vi "Spectral Leakage & window effect.vi"() -> ()   [LabVIEW 2009]
uses:
  <vilib>/Analysis/2dsp.llb/Power Spectrum (DBL).vi
  <vilib>/Analysis/4window.llb/Hanning Window (DBL).vi
  <vilib>/Analysis/4window.llb/Hamming Window (DBL).vi
  <vilib>/Analysis/4window.llb/Triangle Window (DBL).vi
  <vilib>/Analysis/4window.llb/Exponential Window (DBL).vi
  <vilib>/Analysis/4window.llb/Kaiser-Bessel Window (DBL).vi
  <vilib>/Analysis/NI_AALBase.lvlib
  <vilib>/Analysis/NI_AALPro.lvlib
panel:
  out "?":bool
  out "Time domain waveform with periodic repetition":dbl[](graph)=[0.0, 0.06279051952931337, 0.12533323356430423, 0.18738131458572463, 0.24868988716485477, 0.3090169943749474, 0.3681245526846779, 0.42577929156507266, 0.48175367410171527, 0.5358267949789965, 0.5877852522924731, 0.6374239897486896, 0.6845471059286886, 0.7289686274214116, 0.7705132427757893, 0.8090169943749475, 0.8443279255020151, 0.8763066800438636, 0.9048270524660195, 0.9297764858882513, 0.9510565162951535, 0.9685831611286311, 0.9822872507286887, 0.9921147013144779, 0.9980267284282716, 1.0, 0.9980267284282716, 0.9921147013144779, 0.9822872507286887, 0.9685831611286312, 0.9510565162951536, 0.9297764858882515, 0.9048270524660196, 0.8763066800438636, 0.8443279255020151, 0.8090169943749475, 0.7705132427757893, 0.7289686274214116, 0.6845471059286887, 0.6374239897486897, 0.5877852522924732, 0.5358267949789967, 0.4817536741017154, 0.42577929156507277, 0.3681245526846781, 0.3090169943749475, 0.2486898871648549, 0.18738131458572474, 0.12533323356430437, 0.0627905195293135, 1.2354483755472323e-16, -0.06279051952931325, -0.12533323356430412, -0.1873813145857245, -0.24868988716485466, -0.3090169943749473, -0.3681245526846778, -0.42577929156507255, -0.48175367410171516, -0.5358267949789965, -0.587785252292473, -0.6374239897486896, -0.6845471059286886, -0.7289686274214114, -0.7705132427757891, -0.8090169943749473, -0.844327925502015, -0.8763066800438635, -0.9048270524660195, -0.9297764858882513, -0.9510565162951535, -0.9685831611286311, -0.9822872507286886, -0.9921147013144778, -0.9980267284282716, -1.0, -0.9980267284282716, -0.9921147013144779, -0.9822872507286887, -0.9685831611286312, -0.9510565162951536, -0.9297764858882515, -0.9048270524660196, -0.8763066800438637, -0.8443279255020152, -0.8090169943749476, -0.7705132427757894, -0.7289686274214117, -0.6845471059286888, -0.6374239897486899, -0.5877852522924734, -0.5358267949789968, -0.4817536741017155, -0.4257792915650729, -0.3681245526846782, -0.3090169943749477, -0.24868988716485502, -0.18738131458572488, -0.12533323356430448, -0.06279051952931362, 0.0, 0.06279051952931337, 0.12533323356430423, 0.18738131458572463, 0.24868988716485477, 0.3090169943749474, 0.3681245526846779, 0.42577929156507266, 0.48175367410171527, 0.5358267949789965, 0.5877852522924731, 0.6374239897486896, 0.6845471059286886, 0.7289686274214116, 0.7705132427757893, 0.8090169943749475, 0.8443279255020151, 0.8763066800438636, 0.9048270524660195, 0.9297764858882513, 0.9510565162951535, 0.9685831611286311, 0.9822872507286887, 0.9921147013144779, 0.9980267284282716, 1.0, 0.9980267284282716, 0.9921147013144779, 0.9822872507286887, 0.9685831611286312, 0.9510565162951536, 0.9297764858882515, 0.9048270524660196, 0.8763066800438636, 0.8443279255020151, 0.8090169943749475, 0.7705132427757893, 0.7289686274214116, 0.6845471059286887, 0.6374239897486897, 0.5877852522924732, 0.5358267949789967, 0.4817536741017154, 0.42577929156507277, 0.3681245526846781, 0.3090169943749475, 0.2486898871648549, 0.18738131458572474, 0.12533323356430437, 0.0627905195293135, 1.2354483755472323e-16, -0.06279051952931325, -0.12533323356430412, -0.1873813145857245, -0.24868988716485466, -0.3090169943749473, -0.3681245526846778, -0.42577929156507255, -0.48175367410171516, -0.5358267949789965, -0.587785252292473, -0.6374239897486896, -0.6845471059286886, -0.7289686274214114, -0.7705132427757891, -0.8090169943749473, -0.844327925502015, -0.8763066800438635, -0.9048270524660195, -0.9297764858882513, -0.9510565162951535, -0.9685831611286311, -0.9822872507286886, -0.9921147013144778, -0.9980267284282716, -1.0, -0.9980267284282716, -0.9921147013144779, -0.9822872507286887, -0.9685831611286312, -0.9510565162951536, -0.9297764858882515, -0.9048270524660196, -0.8763066800438637, -0.8443279255020152, -0.8090169943749476, -0.7705132427757894, -0.7289686274214117, -0.6845471059286888, -0.6374239897486899, -0.5877852522924734, -0.5358267949789968, -0.4817536741017155, -0.4257792915650729, -0.3681245526846782, -0.3090169943749477, -0.24868988716485502, -0.18738131458572488, -0.12533323356430448, -0.06279051952931362, 0.0, 0.06279051952931337, 0.12533323356430423, 0.18738131458572463, 0.24868988716485477, 0.3090169943749474, 0.3681245526846779, 0.42577929156507266, 0.48175367410171527, 0.5358267949789965, 0.5877852522924731, 0.6374239897486896, 0.6845471059286886, 0.7289686274214116, 0.7705132427757893, 0.8090169943749475, 0.8443279255020151, 0.8763066800438636, 0.9048270524660195, 0.9297764858882513, 0.9510565162951535, 0.9685831611286311, 0.9822872507286887, 0.9921147013144779, 0.9980267284282716, 1.0, 0.9980267284282716, 0.9921147013144779, 0.9822872507286887, 0.9685831611286312, 0.9510565162951536, 0.9297764858882515, 0.9048270524660196, 0.8763066800438636, 0.8443279255020151, 0.8090169943749475, 0.7705132427757893, 0.7289686274214116, 0.6845471059286887, 0.6374239897486897, 0.5877852522924732, 0.5358267949789967, 0.4817536741017154, 0.42577929156507277, 0.3681245526846781, 0.3090169943749475, 0.2486898871648549, 0.18738131458572474, 0.12533323356430437, 0.0627905195293135, 1.2354483755472323e-16, -0.06279051952931325, -0.12533323356430412, -0.1873813145857245, -0.24868988716485466, -0.3090169943749473, -0.3681245526846778, -0.42577929156507255, -0.48175367410171516, -0.5358267949789965, -0.587785252292473, -0.6374239897486896, -0.6845471059286886, -0.7289686274214114, -0.7705132427757891, -0.8090169943749473, -0.844327925502015, -0.8763066800438635, -0.9048270524660195, -0.9297764858882513, -0.9510565162951535, -0.9685831611286311, -0.9822872507286886, -0.9921147013144778, -0.9980267284282716, -1.0, -0.9980267284282716, -0.9921147013144779, -0.9822872507286887, -0.9685831611286312, -0.9510565162951536, -0.9297764858882515, -0.9048270524660196, -0.8763066800438637, -0.8443279255020152, -0.8090169943749476, -0.7705132427757894, -0.7289686274214117, -0.6845471059286888, -0.6374239897486899, -0.5877852522924734, -0.5358267949789968, -0.4817536741017155, -0.4257792915650729, -0.3681245526846782, -0.3090169943749477, -0.24868988716485502, -0.18738131458572488, -0.12533323356430448, -0.06279051952931362]
  in  "Beta":dbl
  in  "Final value":dbl min=0.0 max=1.0
  in  "WINDOW SELECTION":T1(ring)
  out "Frequency\n Domain (without Nyquist shift)":cluster{dbl[]}[](graph)=[{[-717.9728168160375, -12.041199826559248, -665.4873643647093, -666.5995099029594, -669.1691632658144, -677.6948998948894, -681.0329352713741, -671.6665379094907, -689.1835321816163, -671.0719482760868, -689.2418614836788, -672.621826473416, -701.957270271522, -696.8532852986106, -699.451463656731, -692.8383353860734, -682.2898330103367, -698.4054730062687, -707.0532336610472, -669.1255959463351, -707.2021141139068, -686.286325714701, -709.9481162420018, -722.3894498312288, -680.343553829749, -707.4833793420511, -683.1290877804176, -715.3954757206127, -701.1845387253027, -662.9236503342374, -702.6771685318919, -678.1983559742026, -688.0233871040186, -694.8478727739428, -682.6498613386614, -710.6827112012634, -685.7413183239719, -695.7380708290177, -702.9080625621561, -687.1093940743207, -701.1813999614833, -687.5117716388966, -683.6478766075195, -693.9397092458923, -696.0469234579446, -697.7718028900654, -700.095895469833, -691.0074396642474, -694.6133804341445, -703.2922193198955, -697.7736277833116, -703.2922193198955, -694.6133804341445, -691.0074396642474, -700.095895469833, -697.7718028900654, -696.0469234579446, -693.9397092458923, -683.6478766075195, -687.5117716388966, -701.1813999614833, -687.1093940743207, -702.9080625621561, -695.7380708290177, -685.7413183239719, -710.6827112012634, -682.6498613386614, -694.8478727739428, -688.0233871040186, -678.1983559742026, -702.6771685318919, -662.9236503342374, -701.1845387253027, -715.3954757206127, -683.1290877804176, -707.4833793420511, -680.343553829749, -722.3894498312288, -709.9481162420018, -686.286325714701, -707.2021141139068, -669.1255959463351, -707.0532336610472, -698.4054730062687, -682.2898330103367, -692.8383353860734, -699.451463656731, -696.8532852986106, -701.957270271522, -672.621826473416, -689.2418614836788, -671.0719482760868, -689.1835321816163, -671.6665379094907, -681.0329352713741, -677.6948998948894, -669.1691632658144, -666.5995099029594, -665.4873643647093, -12.041199826559248]}, {[-662.5234612067311, -24.082399653118497, -36.12359947967774, -686.0391501168739, -674.2650878771286, -705.9966216646466, -682.162384061586, -693.5568602960511, -708.2455189374288, -676.9926374665027, -713.7575746206643, -678.0624747732352, -692.8167424503345, -688.5243172746942, -693.2645231323679, -701.7444563843032, -695.9087779401403, -690.0885198379467, -690.4467642576584, -682.1856808023391, -728.2256383540973, -683.3629541008854, -687.4572822103436, -724.8745272591966, -713.4517040919175, -703.5234323149774, -698.75063890254, -693.7459180991335, -696.0122919812911, -673.7183454293233, -693.9731458975725, -677.0281334674862, -712.0669993234728, -722.7708351339987, -688.1087311691958, -699.2377312537521, -705.1978959578129, -697.4552667133765, -715.643610874567, -694.98626076297, -731.5654873669778, -685.4026578115215, -694.3961609277321, -718.8382831595254, -691.9463362592454, -697.3136367707239, -761.427863621243, -702.8552652123016, -688.0472344934774, -705.6030194961304, -708.6337726784353, -705.6030194961304, -688.0472344934774, -702.8552652123016, -761.427863621243, -697.3136367707239, -691.9463362592454, -718.8382831595254, -694.3961609277321, -685.4026578115215, -731.5654873669778, -694.98626076297, -715.643610874567, -697.4552667133765, -705.1978959578129, -699.2377312537521, -688.1087311691958, -722.7708351339987, -712.0669993234728, -677.0281334674862, -693.9731458975725, -673.7183454293233, -696.0122919812911, -693.7459180991335, -698.75063890254, -703.5234323149774, -713.4517040919175, -724.8745272591966, -687.4572822103436, -683.3629541008854, -728.2256383540973, -682.1856808023391, -690.4467642576584, -690.0885198379467, -695.9087779401403, -701.7444563843032, -693.2645231323679, -688.5243172746942, -692.8167424503345, -678.0624747732352, -713.7575746206643, -676.9926374665027, -708.2455189374288, -693.5568602960511, -682.162384061586, -705.9966216646466, -674.2650878771286, -686.0391501168739, -36.12359947967774, -24.082399653118497]}]
  out "Time domain waveform":dbl[](graph)=[0.0, 0.06279051952931337, 0.12533323356430423, 0.18738131458572463, 0.24868988716485477, 0.3090169943749474, 0.3681245526846779, 0.42577929156507266, 0.48175367410171527, 0.5358267949789965, 0.5877852522924731, 0.6374239897486896, 0.6845471059286886, 0.7289686274214116, 0.7705132427757893, 0.8090169943749475, 0.8443279255020151, 0.8763066800438636, 0.9048270524660195, 0.9297764858882513, 0.9510565162951535, 0.9685831611286311, 0.9822872507286887, 0.9921147013144779, 0.9980267284282716, 1.0, 0.9980267284282716, 0.9921147013144779, 0.9822872507286887, 0.9685831611286312, 0.9510565162951536, 0.9297764858882515, 0.9048270524660196, 0.8763066800438636, 0.8443279255020151, 0.8090169943749475, 0.7705132427757893, 0.7289686274214116, 0.6845471059286887, 0.6374239897486897, 0.5877852522924732, 0.5358267949789967, 0.4817536741017154, 0.42577929156507277, 0.3681245526846781, 0.3090169943749475, 0.2486898871648549, 0.18738131458572474, 0.12533323356430437, 0.0627905195293135, 1.2354483755472323e-16, -0.06279051952931325, -0.12533323356430412, -0.1873813145857245, -0.24868988716485466, -0.3090169943749473, -0.3681245526846778, -0.42577929156507255, -0.48175367410171516, -0.5358267949789965, -0.587785252292473, -0.6374239897486896, -0.6845471059286886, -0.7289686274214114, -0.7705132427757891, -0.8090169943749473, -0.844327925502015, -0.8763066800438635, -0.9048270524660195, -0.9297764858882513, -0.9510565162951535, -0.9685831611286311, -0.9822872507286886, -0.9921147013144778, -0.9980267284282716, -1.0, -0.9980267284282716, -0.9921147013144779, -0.9822872507286887, -0.9685831611286312, -0.9510565162951536, -0.9297764858882515, -0.9048270524660196, -0.8763066800438637, -0.8443279255020152, -0.8090169943749476, -0.7705132427757894, -0.7289686274214117, -0.6845471059286888, -0.6374239897486899, -0.5877852522924734, -0.5358267949789968, -0.4817536741017155, -0.4257792915650729, -0.3681245526846782, -0.3090169943749477, -0.24868988716485502, -0.18738131458572488, -0.12533323356430448, -0.06279051952931362]
  in  "Cycles":dbl(knob)=1.0 scale=0.0..10.0 scale format="%#.2p"
  in  "stop":bool
  out "Frequency\n Domain (with Nyquist shift)":cluster{dbl[]}[](graph)=[{[-697.7736277833116, -703.2922193198955, -694.6133804341445, -691.0074396642474, -700.095895469833, -697.7718028900654, -696.0469234579446, -693.9397092458923, -683.6478766075195, -687.5117716388966, -701.1813999614833, -687.1093940743207, -702.9080625621561, -695.7380708290177, -685.7413183239719, -710.6827112012634, -682.6498613386614, -694.8478727739428, -688.0233871040186, -678.1983559742026, -702.6771685318919, -662.9236503342374, -701.1845387253027, -715.3954757206127, -683.1290877804176, -707.4833793420511, -680.343553829749, -722.3894498312288, -709.9481162420018, -686.286325714701, -707.2021141139068, -669.1255959463351, -707.0532336610472, -698.4054730062687, -682.2898330103367, -692.8383353860734, -699.451463656731, -696.8532852986106, -701.957270271522, -672.621826473416, -689.2418614836788, -671.0719482760868, -689.1835321816163, -671.6665379094907, -681.0329352713741, -677.6948998948894, -669.1691632658144, -666.5995099029594, -665.4873643647093, -12.041199826559248, -717.9728168160375, -12.041199826559248, -665.4873643647093, -666.5995099029594, -669.1691632658144, -677.6948998948894, -681.0329352713741, -671.6665379094907, -689.1835321816163, -671.0719482760868, -689.2418614836788, -672.621826473416, -701.957270271522, -696.8532852986106, -699.451463656731, -692.8383353860734, -682.2898330103367, -698.4054730062687, -707.0532336610472, -669.1255959463351, -707.2021141139068, -686.286325714701, -709.9481162420018, -722.3894498312288, -680.343553829749, -707.4833793420511, -683.1290877804176, -715.3954757206127, -701.1845387253027, -662.9236503342374, -702.6771685318919, -678.1983559742026, -688.0233871040186, -694.8478727739428, -682.6498613386614, -710.6827112012634, -685.7413183239719, -695.7380708290177, -702.9080625621561, -687.1093940743207, -701.1813999614833, -687.5117716388966, -683.6478766075195, -693.9397092458923, -696.0469234579446, -697.7718028900654, -700.095895469833, -691.0074396642474, -694.6133804341445, -703.2922193198955]}, {[-708.6337726784353, -705.6030194961304, -687.0278840301485, -702.8552652123016, -761.427863621243, -697.3136367707239, -691.9463362592454, -718.8382831595254, -694.3961609277321, -685.4026578115215, -731.5654873669778, -694.98626076297, -715.643610874567, -697.4552667133765, -705.1978959578129, -699.2377312537521, -688.1087311691958, -722.7708351339987, -712.0669993234728, -677.0281334674862, -693.9731458975725, -673.7183454293233, -696.0122919812911, -693.7459180991335, -698.75063890254, -703.5234323149774, -713.4517040919175, -724.8745272591966, -687.4572822103436, -683.3629541008854, -728.2256383540973, -682.1856808023391, -690.4467642576584, -690.0885198379467, -695.9087779401403, -701.7444563843032, -693.2645231323679, -688.5243172746942, -692.8167424503345, -678.0624747732352, -713.7575746206643, -676.9926374665027, -708.2455189374288, -693.5568602960511, -682.162384061586, -705.9966216646466, -674.2650878771286, -686.0391501168739, -36.12359947967774, -24.082399653118497, -662.5234612067311, -24.082399653118497, -36.12359947967774, -686.0391501168739, -674.2650878771286, -705.9966216646466, -682.162384061586, -693.5568602960511, -708.2455189374288, -676.9926374665027, -713.7575746206643, -678.0624747732352, -692.8167424503345, -688.5243172746942, -693.2645231323679, -701.7444563843032, -695.9087779401403, -690.0885198379467, -690.4467642576584, -682.1856808023391, -728.2256383540973, -683.3629541008854, -687.4572822103436, -724.8745272591966, -713.4517040919175, -703.5234323149774, -698.75063890254, -693.7459180991335, -696.0122919812911, -673.7183454293233, -693.9731458975725, -677.0281334674862, -712.0669993234728, -722.7708351339987, -688.1087311691958, -699.2377312537521, -705.1978959578129, -697.4552667133765, -715.643610874567, -694.98626076297, -731.5654873669778, -685.4026578115215, -694.3961609277321, -718.8382831595254, -691.9463362592454, -697.3136367707239, -761.427863621243, -702.8552652123016, -687.0278840301485, -705.6030194961304]}]
  # "The DFT/FFT assumes that the finite time waveform that you obtain is one period of a periodic signal that exist for all\ntime. This assumption of periodicity could result in discontinuities  in the periodic signal  & give rise to spectral leakage,\nwhereby the energy  at a  particular frequency leaks throughout the spectrum.  To reduce  the spectral  leakage, the \nfinite time waveform is multiplied by a \"window\" function."
  # "SPECTRAL LEAKAGE"
  # "WINDOW CHARACTERISTICS"
  # "EXPONENTIAL"
  # "db"
  # "db"
  # "KAISER-BESSEL"
  # "POWER SPECTRUM"
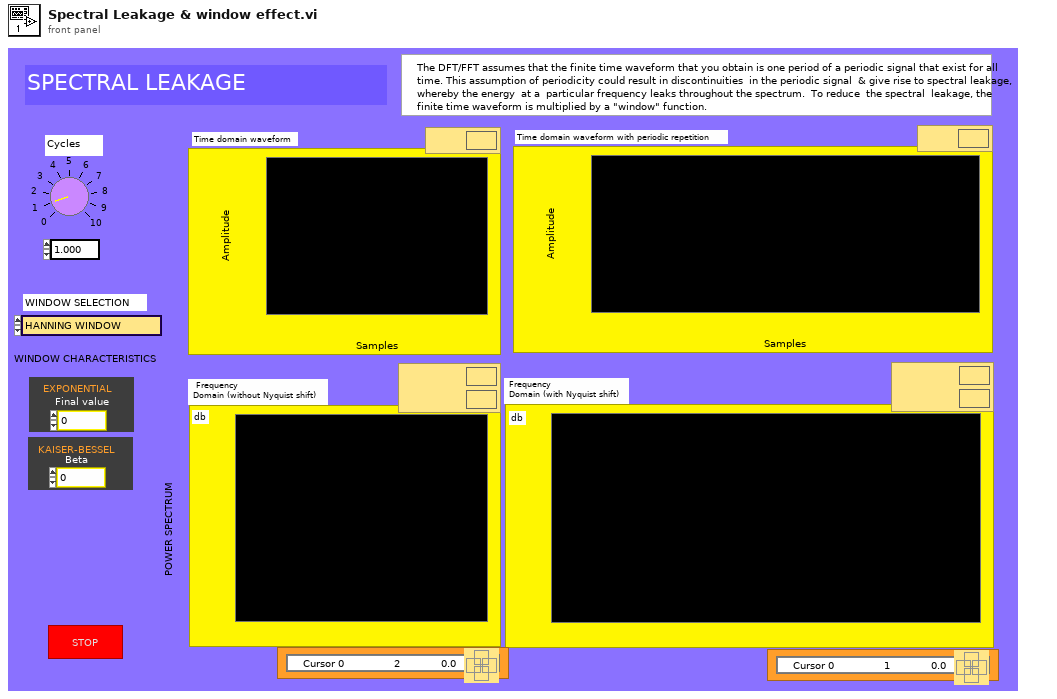
[diagram p1: front panel]
types:
  T1 = enum16{"HANNING WINDOW", "HAMMING WINDOW", "TRIANGLE WINDOW", "EXPONENTIAL WINDOW", "KAISER-BESSEL WINDOW"}
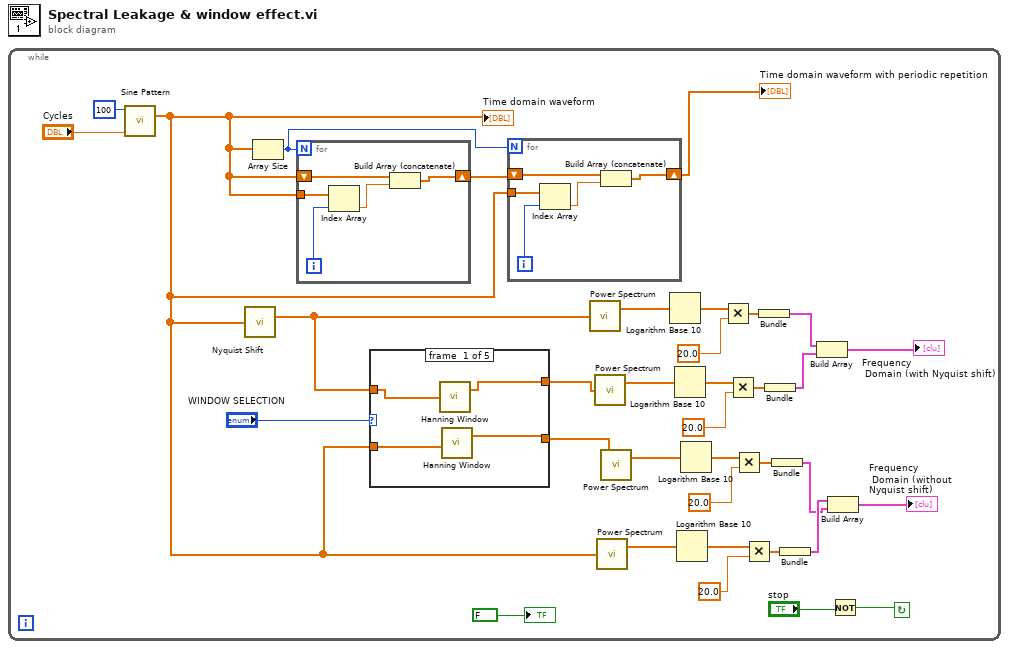
[diagram p0: block diagram]
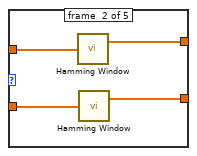
[diagram p2: hidden frame]
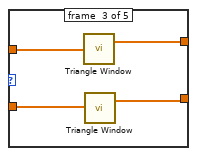
[diagram p3: hidden frame]
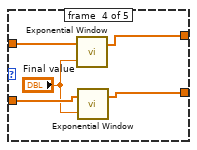
[diagram p4: hidden frame]
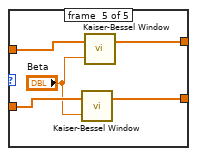
[diagram p5: hidden frame]
diagram:
  n1 = while {
    stop <- w34 continue-if-true
    n2 = call <vilib>:"Sine Pattern.vi"("cycles"="Cycles", "samples"=100) -> ("Sinusoidal Pattern"=w2:dbl[])  [unwired: 2 in, 1 out]
    "Time domain waveform" <- w2
    n3 = call "Nyquist Shift.vi"("X"=w2) -> ("Nyquist Shift{X}"=w24:dbl[])
    n4 = Array Size(array=w2) -> (size(s)=w5:i32)
    n5 = for {
      N: w5 -> [_]
      tunnel: w2 -> [w45]
      shift-right: [w42] -> w3
      shift-left: w2 -> [w41]
      i -> [w44]
      n6 = Index Array(array=w45, index=w44) -> (element=w43:dbl)
      n7 = Build Array (concatenate)(w41, w43) -> (w42:dbl[])
    }
    n8 = case shown="\"EXPONENTIAL WINDOW\"" "WINDOW SELECTION" {
      tunnel: w24 -> [w49 w52 w57 w62 w66]
      tunnel: w2 -> [w48 w53 w56 w60 w64]
      tunnel: [w46 w51 w55 w61 w67] -> w9
      tunnel: [w47 w50 w54 w59 w65] -> w8
      frame #0 {
        n9 = call-poly <vilib>:"Hanning Window.vi"("X"=w49) -> ("Windowed X"=w46:dbl[])  [unwired: 1 out]
        n10 = call-poly <vilib>:"Hanning Window.vi"("X"=w48) -> ("Windowed X"=w47:dbl[])  [unwired: 1 out]
      }
      frame #1 {
        n11 = call-poly <vilib>:"Hamming Window.vi"("X"=w52) -> ("Windowed X"=w51:dbl[])  [unwired: 1 out]
        n12 = call-poly <vilib>:"Hamming Window.vi"("X"=w53) -> ("Windowed X"=w50:dbl[])  [unwired: 1 out]
      }
      frame #2 {
        n13 = call-poly <vilib>:"Triangle Window.vi"("X"=w57) -> ("Windowed X"=w55:dbl[])  [unwired: 1 out]
        n14 = call-poly <vilib>:"Triangle Window.vi"("X"=w56) -> ("Windowed X"=w54:dbl[])  [unwired: 1 out]
      }
      frame #3 {
        n15 = call-poly <vilib>:"Exponential Window.vi"("final value"="Final value", "X"=w62) -> ("Windowed X"=w61:dbl[])  [unwired: 1 out]
        n16 = call-poly <vilib>:"Exponential Window.vi"("final value"="Final value", "X"=w60) -> ("Windowed X"=w59:dbl[])  [unwired: 1 out]
      }
      frame #4 {
        n17 = call-poly <vilib>:"Kaiser-Bessel Window.vi"("beta"="Beta", "X"=w64) -> ("Windowed X"=w65:dbl[])  [unwired: 1 out]
        n18 = call-poly <vilib>:"Kaiser-Bessel Window.vi"("beta"="Beta", "X"=w66) -> ("Windowed X"=w67:dbl[])  [unwired: 1 out]
      }
    }
    n19 = for {
      N: w5 -> [_]
      tunnel: w2 -> [w40]
      shift-right: [w37] -> w4
      shift-left: w3 -> [w36]
      i -> [w39]
      n20 = Index Array(array=w40, index=w39) -> (element=w38:dbl)
      n21 = Build Array (concatenate)(w36, w38) -> (w37:dbl[])
    }
    "Time domain waveform with periodic repetition" <- w4
    n22 = call-poly <vilib>:"Power Spectrum.vi"("X"=w24) -> ("Power Spectrum"=w31:dbl[])  [unwired: 1 out]
    n23 = call-poly <vilib>:"Power Spectrum.vi"("X"=w9) -> ("Power Spectrum"=w21:dbl[])  [unwired: 1 out]
    n24 = call-poly <vilib>:"Power Spectrum.vi"("X"=w2) -> ("Power Spectrum"=w26:dbl[])  [unwired: 1 out]
    n25 = call-poly <vilib>:"Power Spectrum.vi"("X"=w8) -> ("Power Spectrum"=w20:dbl[])  [unwired: 1 out]
    n26 = Logarithm Base 10(1:w31) -> (0:w30:dbl[])
    n27 = Logarithm Base 10(1:w21) -> (0:w22:dbl[])
    n28 = Logarithm Base 10(1:w26) -> (0:w27:dbl[])
    n29 = Logarithm Base 10(1:w20) -> (0:w19:dbl[])
    n30 = Multiply(x=w30, y=20.0) -> (x*y=w17:dbl[])
    n31 = Multiply(x=w22, y=20.0) -> (x*y=w14:dbl[])
    n32 = Multiply(x=w19, y=20.0) -> (x*y=w15:dbl[])
    n33 = Multiply(x=w27, y=20.0) -> (x*y=w16:dbl[])
    n34 = Bundle(w17) -> (w12:cluster{dbl[]})  [unwired: 1 in]
    n35 = Bundle(w14) -> (w13:cluster{dbl[]})  [unwired: 1 in]
    n36 = Bundle(w15) -> (w6:cluster{dbl[]})  [unwired: 1 in]
    n37 = Bundle(w16) -> (w7:cluster{dbl[]})  [unwired: 1 in]
    n38 = Build Array(w12, w13) -> (→"Frequency\n Domain (with Nyquist shift)":cluster{dbl[]}[])
    n39 = Build Array(w7, w6) -> (→"Frequency\n Domain (without Nyquist shift)":cluster{dbl[]}[])
    n40 = Not(x="stop") -> (.not. x?=w34:bool)
    "?" <- FALSE
  }
